vi "Encoders.vi"(2 "Wheel":T1(ring), 3 "Reset All":bool) -> (0 "Avg Absolute Rate":dbl, 1 "Avg Absolute Distance":dbl)   [LabVIEW 2013]
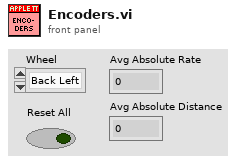
[diagram p1: front panel]
types:
  T1 = enum16{"Back Left", "Back Right", "Front Left", "Front Right"}
  T2 = typedef "WPI_EncoderDevRef.ctl" = cluster{"DevStatus":errorcluster, "EncoderIndex":T3, "CounterIndex":T4, "DistancePerCount":dbl, "Decoding Type":T5}
  T3 = typedef "FPGA_EncoderIdx.ctl" = enum8{"Enc 0", "Enc 1", "Enc 2", "Enc 3", "Invalid"}
  T4 = typedef "FPGA_CounterCtrSystemIndex.ctl" = enum8{"Ctr 0", "Ctr 1", "Ctr 2", "Ctr 3", "Ctr 4", "Ctr 5", "Ctr 6", "Ctr 7", "Invalid"}
  T5 = typedef "WPI_EncoderType.ctl" = enum16{"1x", "2x", "4x"}
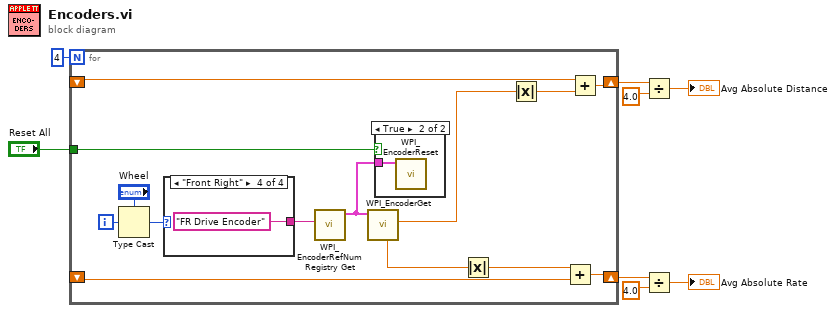
[diagram p0: block diagram]
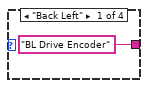
[diagram p3: hidden frame]
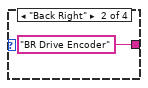
[diagram p4: hidden frame]
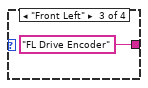
[diagram p5: hidden frame]
diagram:
  n1 = for {
    N: 4 -> [_]
    shift-right: [w19] -> w2
    shift-left: _ -> [w18]
    tunnel: "Reset All" -> [w16]
    shift-right: [w12] -> w6
    shift-left: _ -> [w11]
    i -> [w22]
    n2 = Type Cast(type="Wheel", x=w22) -> (*(type *) &x=w15:T1)
    n3 = case shown="\"Front Right\"" w15 {
      tunnel: ["BL Drive Encoder" ("refnum name") "BR Drive Encoder" ("refnum name") "FL Drive Encoder" ("refnum name") "FR Drive Encoder" ("refnum name")] -> w20
      frame "Back Left" {
      }
      frame "Back Right" {
      }
      frame "Front Left" {
      }
      frame "Front Right" {
      }
    }
    n4 = call <vilib>:"WPI_EncoderRefNum Registry Get.vi"("refnum name"=w20) -> ("EncoderDevRef"=w17:T2)  [unwired: 9 in, 1 out]
    n5 = call <vilib>:"WPI_EncoderGet.vi"("EncoderDevRef"=w17) -> ("Distance"=w9:dbl, "Rate"=w10:dbl)  [unwired: 5 in, 4 out]
    n6 = case shown="True" w16 {
      tunnel: w17 -> [_ w23]
      frame False {
      }
      frame True {
        n7 = call <vilib>:"WPI_EncoderReset.vi"("EncoderDevRef"=w23) -> ()  [unwired: 9 in, 2 out]
      }
    }
    n8 = Absolute Value(x=w10) -> (abs(x)=w14:dbl)
    n9 = Absolute Value(x=w9) -> (abs(x)=w13:dbl)
    n10 = Add(x=w14, y=w18) -> (x+y=w19:dbl)
    n11 = Add(x=w11, y=w13) -> (x+y=w12:dbl)
  }
  n12 = Divide(x=w6, y=4.0) -> (x/y=→"Avg Absolute Distance":dbl)
  n13 = Divide(x=w2, y=4.0) -> (x/y=→"Avg Absolute Rate":dbl)
